vi "onRetrieveResults.vi"(8 "error in (no error)":errorcluster, 10 "Filter":T1=enum."passed", 11 "Pips.TestResults in":refnum<class "Pips.TestResults.lvclass">) -> (0 "error out":errorcluster, 2 "Matrix":bool[][](array[boolean]), 3 "Pips.TestResults out":refnum<class "Pips.TestResults.lvclass">)   [LabVIEW 2021, in "Banana.Caraya.lvlib" / "Pips.TestResults.lvclass"]
uses:
  Pips.TestResults.lvclass
  Pips.TestResults.lvclass/Pips.TestResults.ctl
  Bananas/Pips/Pips.lvclass
  Bananas/Pips/pip_filter -- enum.ctl
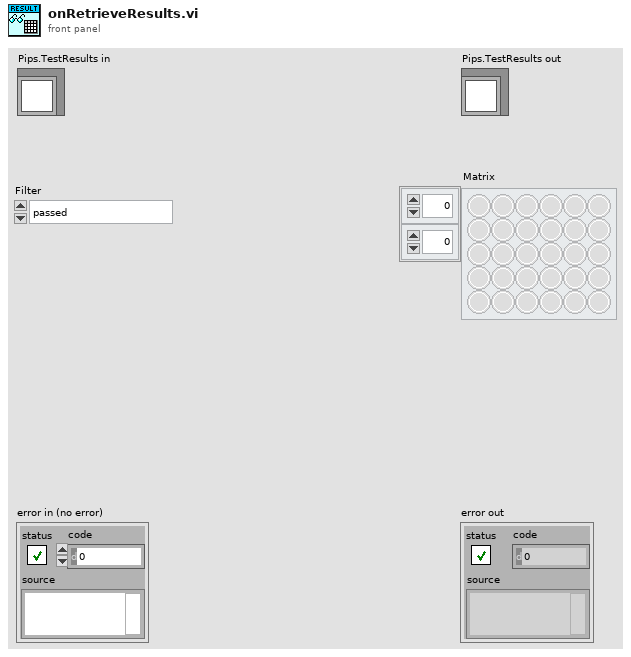
[diagram p1: front panel]
types:
  T1 = typedef "Bananas.lvlib/Pips.lvclass/pip_filter -- enum.ctl" = enum16{"none", "passed", "skipped", "covered", "uncovered"}
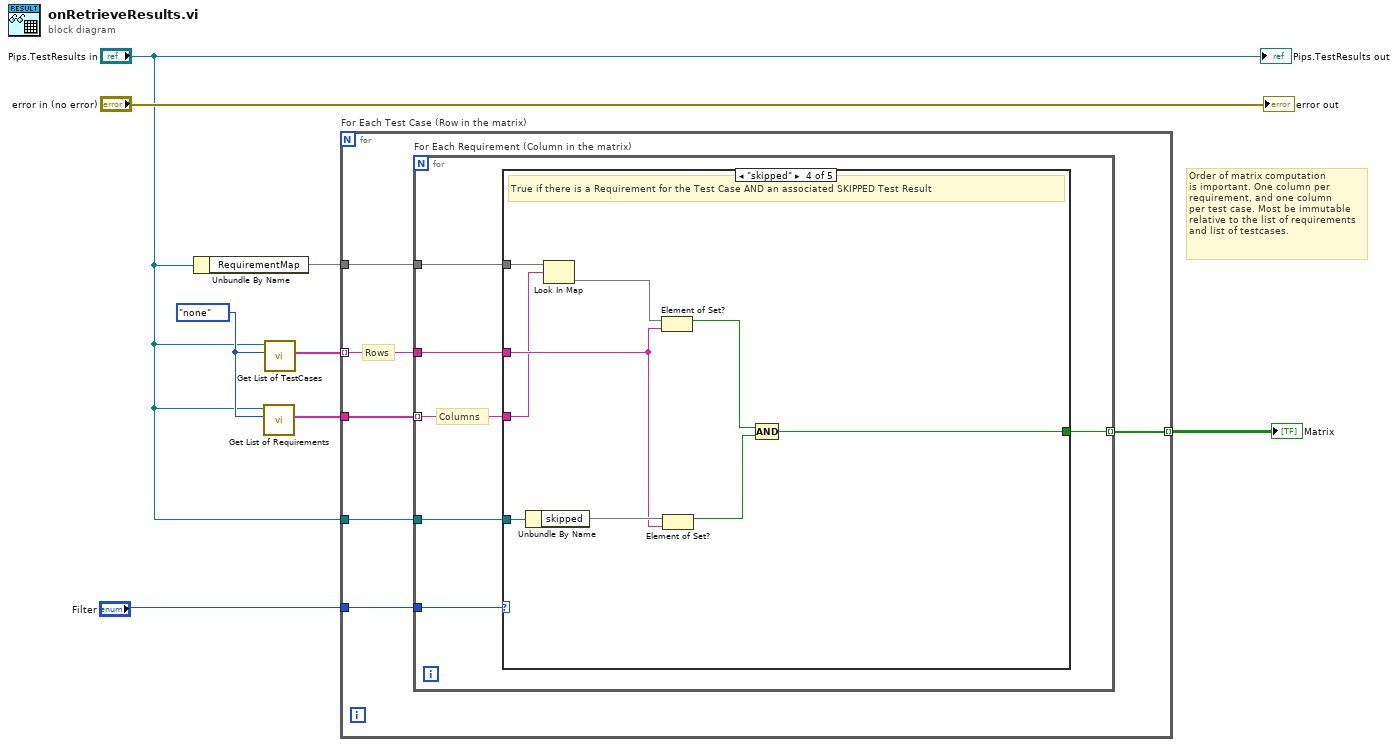
[diagram p0: block diagram]
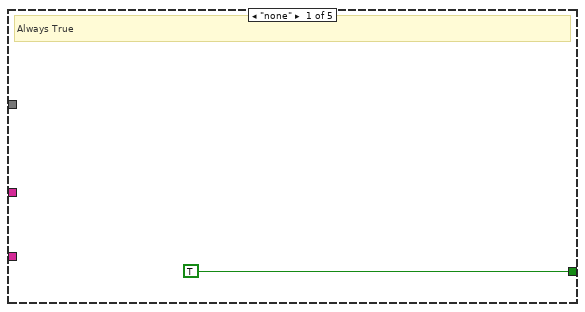
[diagram p2: hidden frame]
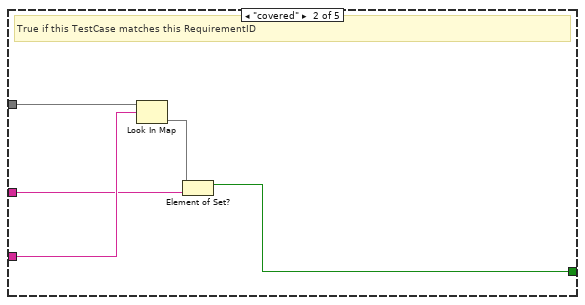
[diagram p3: hidden frame]
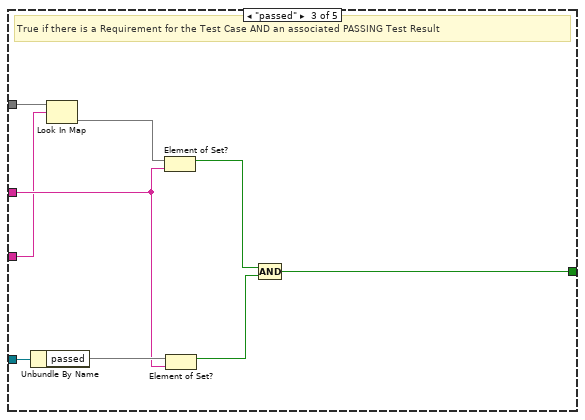
[diagram p4: hidden frame]
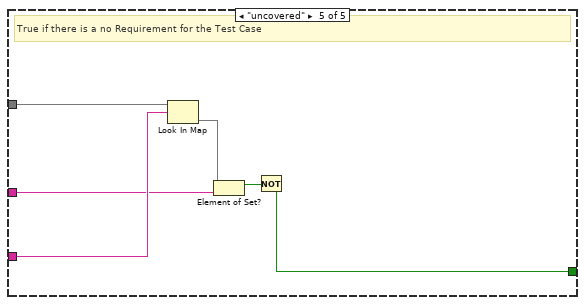
[diagram p5: hidden frame]
diagram:
  w4 = pip_filter_--_enum."none" ("Filter")
  # "Order of matrix computation\nis important. One column per\nrequirement, and one column\nper test case. Most be immutable\nrelative to the list of requirements\nand list of testcases."
  n1 = Unbundle By Name("Pips.TestResults in") -> ("RequirementMap"=w2:map{string, set{string}})
  n2 = call "Get List of Requirements.vi"("Filter"=w4, "Pips in"="Pips.TestResults in") -> ("RequirementIDs"=w3:string[])  [unwired: 7 in, 2 out]
  n3 = call "Get List of TestCases.vi"("Filter"=w4, "Pips in"="Pips.TestResults in") -> ("TestCases"=w5:string[])  [unwired: 7 in, 2 out]
  n4 = for "For Each Test Case (Row in the matrix)" {
    tunnel: "Filter" -> [w14]
    tunnel: w3 -> [w12]
    tunnel: w5 -> [w11] mode=indexing
    tunnel: [w13] -> w6 mode=indexing
    tunnel: w2 -> [w10]
    tunnel: "Pips.TestResults in" -> [w9]
    # "Rows"
    n5 = for "For Each Requirement (Column in the matrix)" {
      tunnel: w14 -> [w20]
      tunnel: [w19] -> w13 mode=indexing
      tunnel: w12 -> [w16] mode=indexing
      tunnel: w11 -> [w18]
      tunnel: w10 -> [w17]
      tunnel: w9 -> [w15]
      # "Columns"
      n6 = case shown="\"skipped\"" w20 {
        tunnel: [TRUE w22 w28 w37 w45] -> w19
        tunnel: w18 -> [_ w23 w31 w39 w47]
        tunnel: w17 -> [_ w26 w34 w40 w49]
        tunnel: w16 -> [_ w25 w27 w36 w48]
        tunnel: w15 -> [_ _ w33 w38 _]
        frame "none" {
          # "Always True"
        }
        frame "covered" {
          # "True if this TestCase matches this RequirementID"
          n7 = Look In Map(map=w26, key=w25) -> (value=w24:set{string})  [unwired: 1 in, 1 out]
          n8 = Element of Set?(10:w23, 11:w24) -> (3:w22:bool)
        }
        frame "passed" {
          # "True if there is a Requirement for the Test Case AND an associated PASSING Test Result"
          n9 = Unbundle By Name(w33) -> ("passed"=w32:set{string})
          n10 = Look In Map(map=w34, key=w27) -> (value=w35:set{string})  [unwired: 1 in, 1 out]
          n11 = Element of Set?(10:w31, 11:w35) -> (3:w30:bool)
          n12 = Element of Set?(10:w31, 11:w32) -> (3:w29:bool)
          n13 = Compound Arithmetic op=AND(w30, w29) -> (w28:bool)
        }
        frame "skipped" {
          # "True if there is a Requirement for the Test Case AND an associated SKIPPED Test Result"
          n14 = Unbundle By Name(w38) -> ("skipped"=w43:set{string})
          n15 = Look In Map(map=w40, key=w36) -> (value=w44:set{string})  [unwired: 1 in, 1 out]
          n16 = Element of Set?(10:w39, 11:w44) -> (3:w42:bool)
          n17 = Element of Set?(10:w39, 11:w43) -> (3:w41:bool)
          n18 = Compound Arithmetic op=AND(w42, w41) -> (w37:bool)
        }
        frame "uncovered" {
          # "True if there is a no Requirement for the Test Case"
          n19 = Look In Map(map=w49, key=w48) -> (value=w50:set{string})  [unwired: 1 in, 1 out]
          n20 = Element of Set?(10:w47, 11:w50) -> (3:w46:bool)
          n21 = Not(x=w46) -> (.not. x?=w45:bool)
        }
      }
    }
  }
  "Matrix" <- w6
  "error out" <- "error in (no error)"
  "Pips.TestResults out" <- "Pips.TestResults in"
